vi "Overview.vi"() -> ()   [LabVIEW 2024]
uses:
  <vilib>/Plug-In SDKs/Clients/Metadata/Operator.ctl
  <vilib>/Plug-In SDKs/Clients/Metadata/Extension.ctl
  <vilib>/Plug-In SDKs/Clients/Metadata/Test Station.ctl
  <vilib>/Plug-In SDKs/Clients/Metadata/Software Item.ctl
  <vilib>/Plug-In SDKs/Clients/Data Store V1/Data Store Client.lvlibp/API/Data Store V1/Test Result.ctl
  <vilib>/Plug-In SDKs/Clients/Metadata/Outcome.ctl
  <vilib>/Plug-In SDKs/Clients/Metadata/Step.ctl
  <vilib>/Plug-In SDKs/Clients/Metadata Store V1/Metadata Store Client.lvlibp/API/Metadata Store V1/Register Schema (String).vi
  <vilib>/Plug-In SDKs/Clients/Metadata Store V1/Metadata Store Client.lvlibp/API/Metadata Store V1/Create Operator.vi
  <vilib>/Plug-In SDKs/Clients/Metadata Store V1/Metadata Store Client.lvlibp/API/Metadata Store V1/Create Test Station.vi
  <vilib>/Plug-In SDKs/Clients/Metadata Store V1/Metadata Store Client.lvlibp/API/Metadata Store V1/Create Software Item.vi
  <vilib>/Plug-In SDKs/Clients/Data Store V1/Data Store Client.lvlibp/API/Data Store V1/Publish Measurement (DBL Analog Waveform).vi
  <vilib>/Plug-In SDKs/Clients/Metadata Store V1/Metadata Store Client.lvlibp/API/Metadata Store V1/Get Operator.vi
  <vilib>/Plug-In SDKs/Clients/Data Store V1/Data Store Client.lvlibp/API/Data Store V1/Read Data from Measurement (DBL Analog Waveform).vi
  <vilib>/Plug-In SDKs/Clients/Metadata Store V1/Metadata Store Client.lvlibp
  <vilib>/Plug-In SDKs/Clients/Data Store V1/Data Store Client.lvlibp
  <vilib>/Plug-In SDKs/Clients/Metadata/NI Metadata Types.lvlib
  <vilib>/measure/NI_MABase.lvlib
panel:
  out "test result id":string
  out "published measurement id":string
  out "schema id":string
  out "Waveform Graph":waveform(dbl)(graph)
  out "log":string
  out "error out":errorcluster
  # "This example publishes a waveform along with metadata and metadata extensions.\nThen it queries for the published data and displays it."
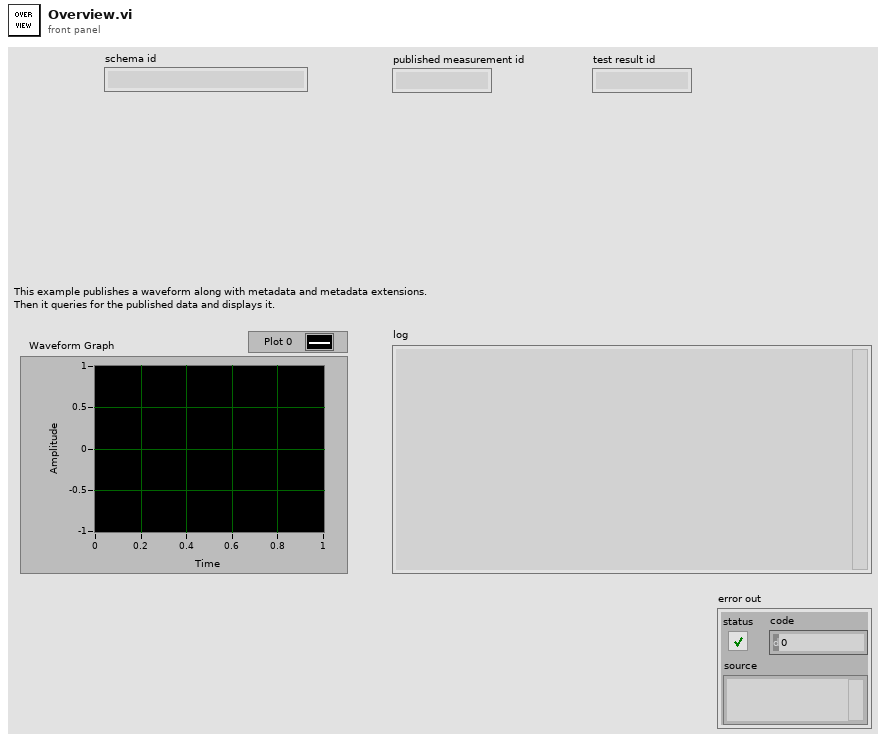
[diagram p1: front panel]
types:
  T1 = enum16{"Register Metadata Schema", "Create Metadata and Test Result", "Publish Data", "Query Published Data"}
  T2 = typedef "NI Metadata Types.lvlib/Extension.ctl" = cluster{"name":string, "value":string}
  T3 = typedef "Data Store Client.lvlibp/Test Result.ctl" = cluster{"test result name":string, "start date time":timestamp, "end date time":timestamp, "outcome":T4, "test result id":string, "uut instance id":string, "operator id":string, "test station id":string, "test description id":string, "software item ids":string[], "hardware item ids":string[], "test adapter ids":string[], "link":string, "extensions":T2[], "schema id":string}
  T4 = typedef "NI Metadata Types.lvlib/Outcome.ctl" = enum32{"Unspecified", "Passed", "Failed", "Indeterminate"}
  T5 = typedef "NI Metadata Types.lvlib/Software Item.ctl" = cluster{"product":string, "version":string, "id":string, "link":string, "extensions":T2[], "schema id":string}
  T6 = typedef "NI Metadata Types.lvlib/Test Station.ctl" = cluster{"test station name":string, "asset identifier":string, "id":string, "link":string, "extensions":T2[], "schema id":string}
  T7 = typedef "NI Metadata Types.lvlib/Operator.ctl" = cluster{"operator name":string, "role":string, "id":string, "link":string, "extensions":T2[], "schema id":string}
  T8 = typedef "NI Metadata Types.lvlib/Step.ctl" = cluster{"step name":string, "step type":string, "start date time":timestamp, "end date time":timestamp, "notes":string, "step id":string, "parent step id":string, "test result id":string, "test id":string, "link":string, "extensions":T2[], "schema id":string}
  T9 = typedef "Data Store Client.lvlibp/Published Measurement.ctl" = cluster{"data moniker":T10, "published conditions":T11[], "published measurement id":string, "test result id":string, "step id":string, "software item ids":string[], "hardware item ids":string[], "test adapter ids":string[], "measurement name":string, "data type":string, "measurement notes":string, "start date time":timestamp, "end date time":timestamp, "outcome":T4, "parametric index":i32, "error information":T12}
  T10 = typedef "Data Store Client.lvlibp/Data Moniker.ctl" = cluster{"service location":string, "data source":string, "data instance":i64}
  T11 = typedef "Data Store Client.lvlibp/Published Condition.ctl" = cluster{"moniker":T10, "published condition id":string, "condition name":string, "condition type":string, "step id":string, "test result id":string}
  T12 = typedef "NI Metadata Types.lvlib/Error Information.ctl" = cluster{"error code":i32, "message":string, "source":string}
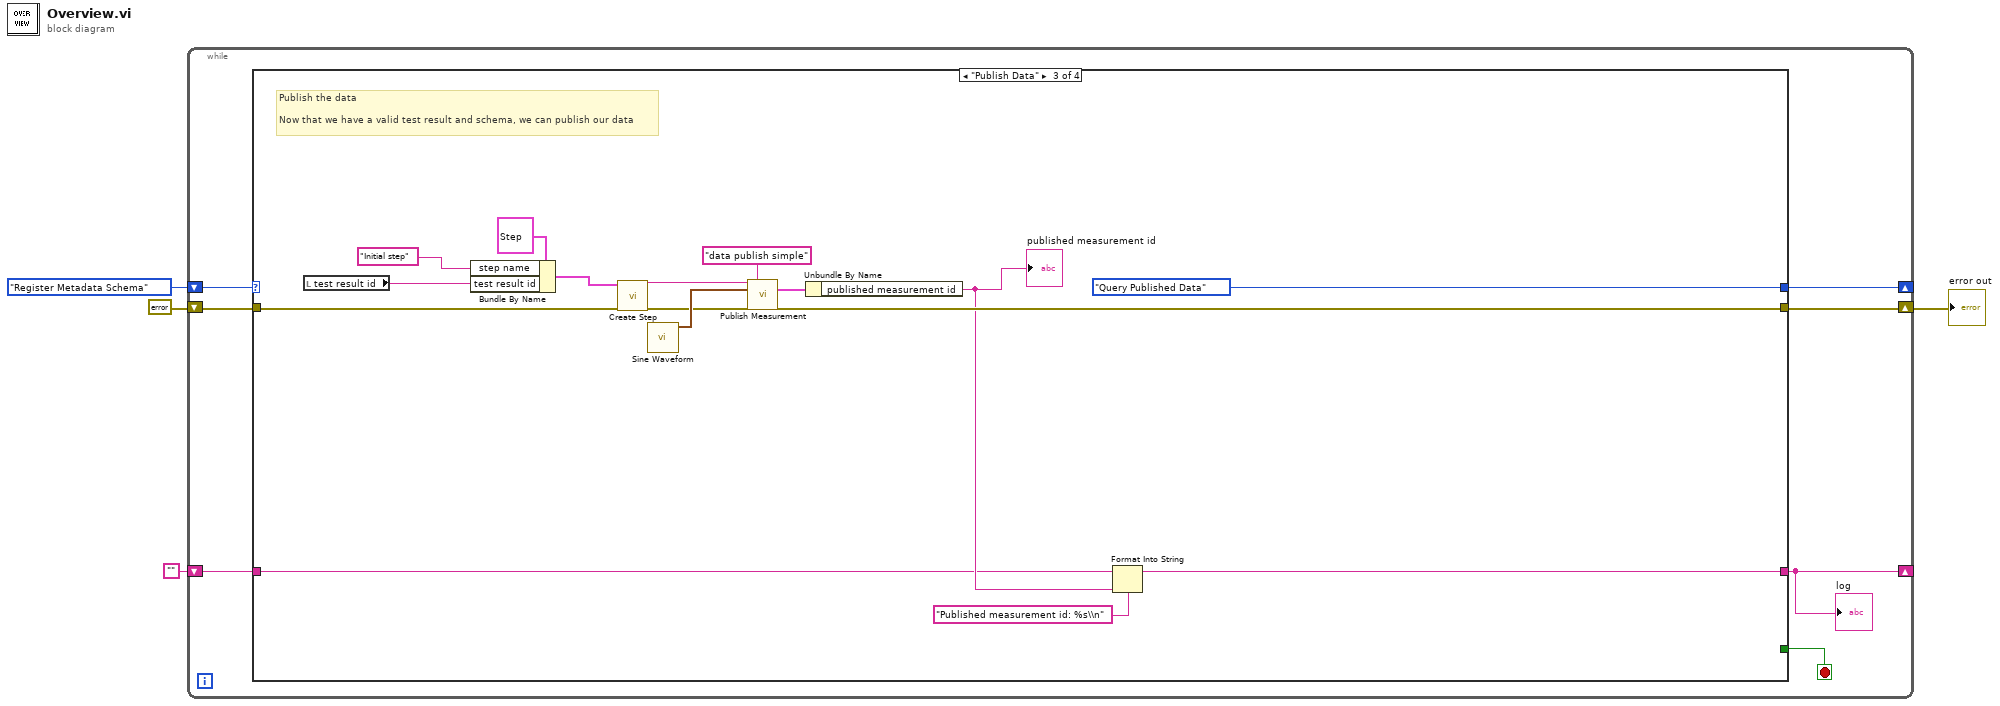
[diagram p0: block diagram]
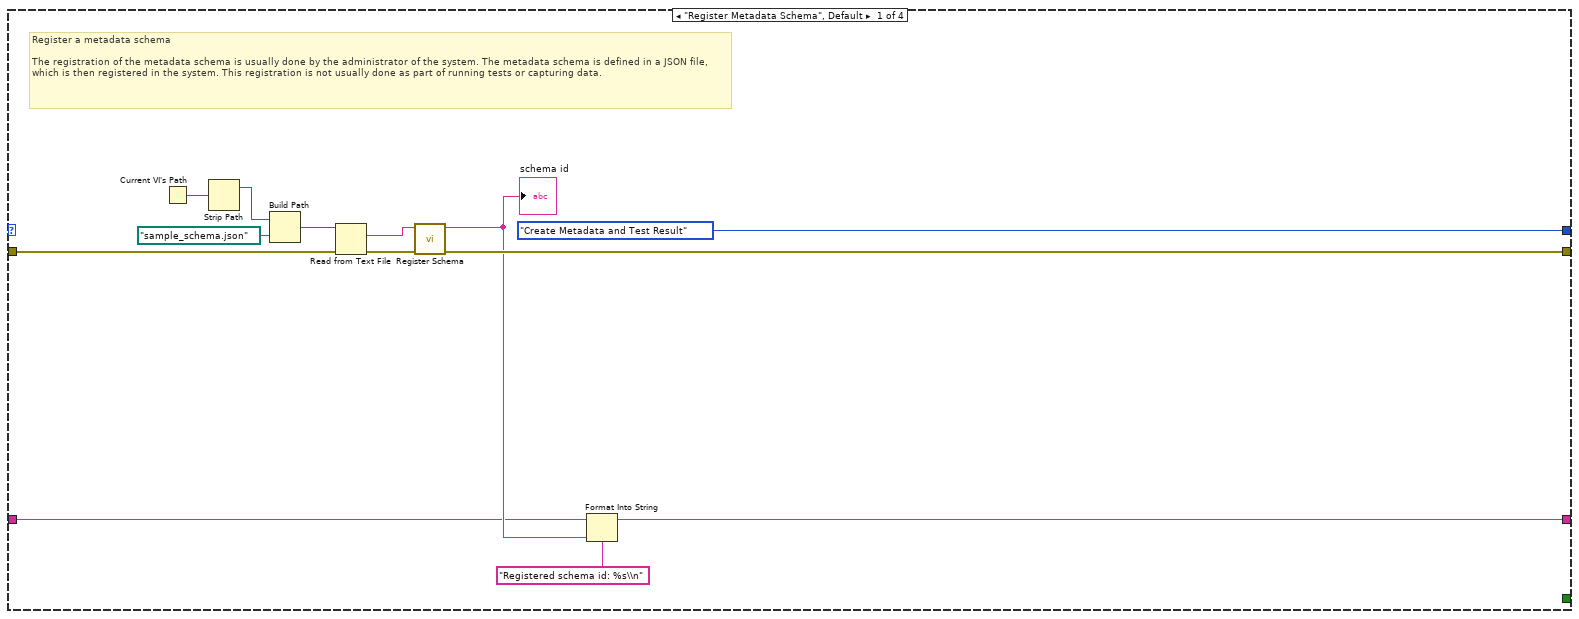
[diagram p2: hidden frame]
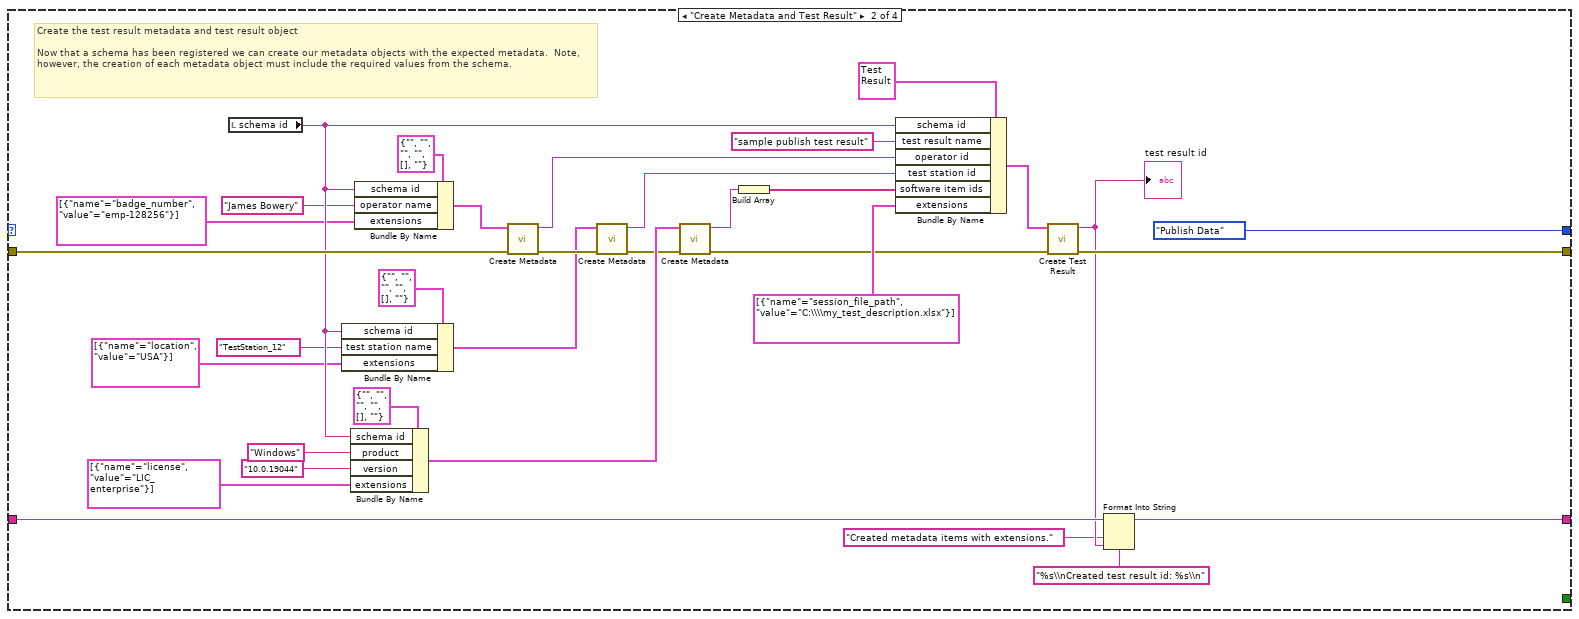
[diagram p3: hidden frame]
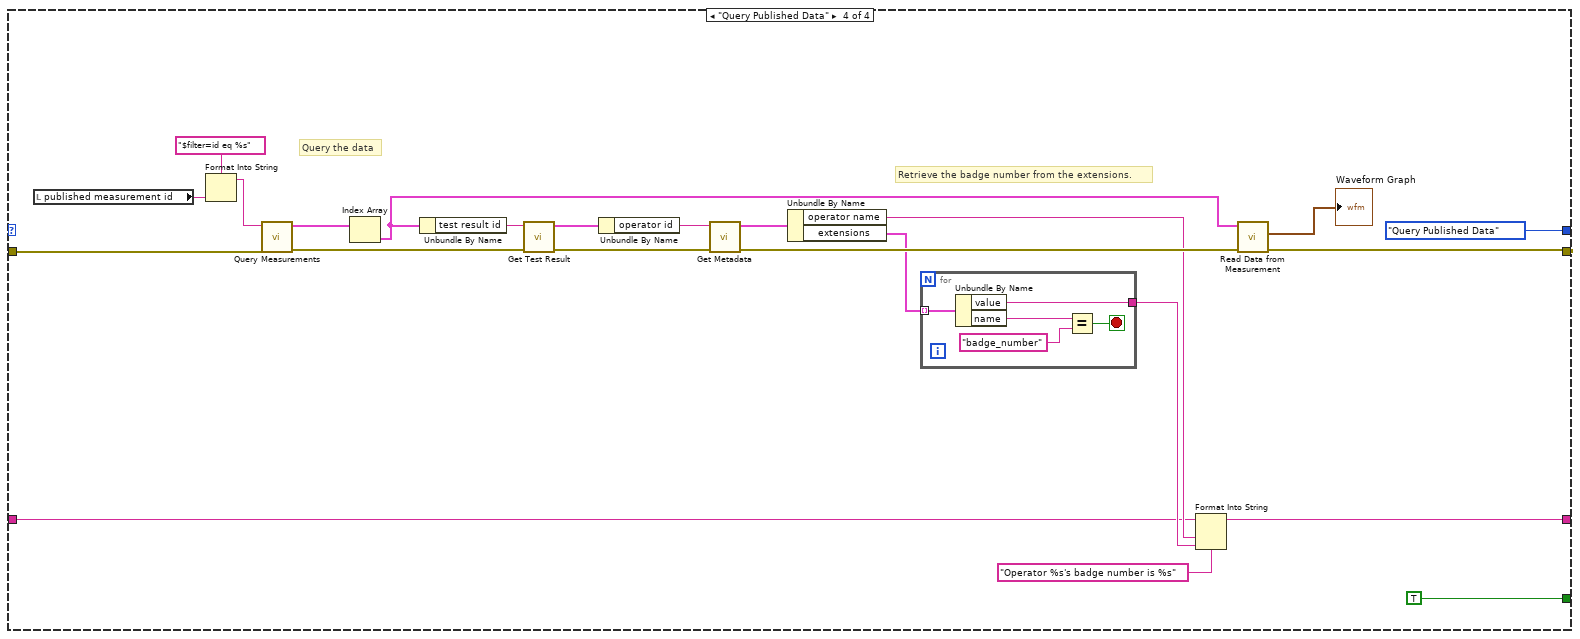
[diagram p4: hidden frame]
diagram:
  n1 = while {
    shift-right: [w7] -> _
    shift-left: T1."Register Metadata Schema" -> [w11]
    shift-right: [w10] -> w2
    shift-left: errorcluster {"status"=FALSE, "code"=0, "source"=""} ("error out") -> [w9]
    shift-right: [w6] -> _
    shift-left: "" ("log") -> [w8]
    stop <- w5 stop-if-true
    n2 = case shown="\"Publish Data\"" w11 {
      tunnel: [w24 w54 w73 w96] -> w10
      tunnel: w9 -> [w23 w55 w61 w95]
      tunnel: [w13 w51 w63 w75] -> w6
      tunnel: w8 -> [w14 w52 w58 w76]
      tunnel: [T1."Create Metadata and Test Result" T1."Publish Data" T1."Query Published Data" T1."Query Published Data"] -> w7
      tunnel: [_ _ _ TRUE] -> w5
      frame "Register Metadata Schema", Default {
        # "Register a metadata schema\n\nThe registration of the metadata schema is usually done by the administrator of the system. The metadata schema is defined in a JSON file, which is then registered in the system. This registration is not usually done as part of running tests or capturing data."
        n3 = Current VI's Path() -> (path=w19:path)
        n4 = Strip Path(path=w19) -> (stripped path=w18:path)  [unwired: 1 out]
        n5 = Build Path(base path=w18, name or relative path=path "sample_schema.json") -> (appended path=w16:path)
        n6 = Read from Text File(file (use dialog)=w16, error in=w23) -> (text=w15:string, error out=w20:errorcluster)  [unwired: 2 in, 2 out]
        n7 = call-poly <vilib>:"Register Schema.vi"("error in"=w20, "schema"=w15) -> ("error out"=w24:errorcluster, "schema id"=w22:string)  [unwired: 8 in]
        "schema id" <- w22
        n8 = Format Into String(format string="Registered schema id: %s\\n", initial string=w14, w22) -> (resulting string=w13:string)  [unwired: 1 in, 1 out]
      }
      frame "Create Metadata and Test Result" {
        # "Create the test result metadata and test result object\n\nNow that a schema has been registered we can create our metadata objects with the expected metadata.  Note, however, the creation of each metadata object must include the required values from the schema."
        n9 = local read "schema id"() -> (w53:string)
        n10 = Bundle By Name(cluster=T6 {"test station name"="", "asset identifier"="", "id"="", "link"="", "extensions"=[], "schema id"=""} ("test station"), "schema id"=w53, "test station name"="TestStation_12", "extensions"=T2[] [{"name"="location", "value"="USA"}]) -> (w25:T6)
        n11 = Bundle By Name(cluster=T5 {"product"="", "version"="", "id"="", "link"="", "extensions"=[], "schema id"=""} ("software item"), "schema id"=w53, "product"="Windows", "version"="10.0.19044", "extensions"=T2[] [{"name"="license", "value"="LIC_enterprise"}]) -> (w29:T5)
        n12 = Bundle By Name(cluster=T7 {"operator name"="", "role"="", "id"="", "link"="", "extensions"=[], "schema id"=""} ("operator metadata"), "schema id"=w53, "operator name"="James Bowery", "extensions"=T2[] [{"name"="badge_number", "value"="emp-128256"}]) -> (w36:T7)
        n13 = call-poly <vilib>:"Create Metadata.vi"("error in"=w55, "operator metadata"=w36) -> ("error out"=w28:errorcluster, "operator id"=w47:string)  [unwired: 8 in]
        n14 = call-poly <vilib>:"Create Metadata.vi"("error in"=w28, "test station"=w25) -> ("error out"=w27:errorcluster, "test station id"=w46:string)  [unwired: 8 in]
        n15 = call-poly <vilib>:"Create Metadata.vi"("error in"=w27, "software item"=w29) -> ("error out"=w26:errorcluster, "software item id"=w45:string)  [unwired: 8 in]
        n16 = Build Array(w45) -> (w42:string[])
        n17 = Bundle By Name(cluster=T3 {"test result name"="", "start date time"=timestamp(0 s since 1904-01-01), "end date time"=timestamp(0 s since 1904-01-01), "outcome"=enum."Unspecified", "test result id"="", "uut instance id"="", "operator id"="", "test station id"="", "test description id"="", "software item ids"=[], "hardware item ids"=[], "test adapter ids"=[], "link"="", "extensions"=[], "schema id"=""} ("test result"), "schema id"=w53, "test result name"="sample publish test result", "operator id"=w47, "test station id"=w46, "software item ids"=w42, "extensions"=T2[] [{"name"="session_file_path", "value"="C:\\\\my_test_description.xlsx"}]) -> (w57:T3)
        n18 = call <vilib>:"Create Test Result.vi"("error in"=w26, "test result"=w57) -> ("error out"=w54:errorcluster, "test result id"=w49:string)  [unwired: 8 in]
        "test result id" <- w49
        n19 = Format Into String(format string="%s\\nCreated test result id: %s\\n", initial string=w52, "Created metadata items with extensions." ("log"), w49) -> (resulting string=w51:string)  [unwired: 1 in, 1 out]
      }
      frame "Publish Data" {
        # "Publish the data\n\nNow that we have a valid test result and schema, we can publish our data"
        n20 = local read "test result id"() -> (w60:string)
        n21 = Bundle By Name(cluster=T8 {"step name"="", "step type"="", "start date time"=timestamp(0 s since 1904-01-01), "end date time"=timestamp(0 s since 1904-01-01), "notes"="", "step id"="", "parent step id"="", "test result id"="", "test id"="", "link"="", "extensions"=[], "schema id"=""} ("step"), "step name"="Initial step", "test result id"=w60) -> (w68:T8)
        n22 = call <vilib>:"Create Step.vi"("error in"=w61, "step"=w68) -> ("error out"=w67:errorcluster, "step id"=w66:string)  [unwired: 8 in]
        n23 = call <vilib>:"Sine Waveform.vi"() -> ("signal out"=w71:waveform(dbl))  [unwired: 10 in, 1 out]
        n24 = call-poly <vilib>:"Publish Measurement.vi"("step id"=w66, "name"="data publish simple", "waveform"=w71, "error in"=w67) -> ("published measurement"=w64:T9, "error out"=w73:errorcluster)  [unwired: 9 in, 1 out]
        n25 = Unbundle By Name(w64) -> ("published measurement id"=w72:string)
        "published measurement id" <- w72
        n26 = Format Into String(format string="Published measurement id: %s\\n", initial string=w58, w72) -> (resulting string=w63:string)  [unwired: 1 in, 1 out]
      }
      frame "Query Published Data" {
        # "Retrieve the badge number from the extensions."
        # "Query the data"
        n27 = local read "published measurement id"() -> (w94:string)
        n28 = Format Into String(format string="$filter=id eq %s", w94) -> (resulting string=w85:string)  [unwired: 2 in, 1 out]
        n29 = call <vilib>:"Query Measurements.vi"("error in"=w95, "odata query"=w85) -> ("error out"=w83:errorcluster, "published measurements"=w84:T9[])  [unwired: 8 in]
        n30 = Index Array(array=w84) -> (element=w77:T9)  [unwired: 1 in]
        n31 = Unbundle By Name(w77) -> ("test result id"=w82:string)
        n32 = call <vilib>:"Get Test Result.vi"("error in"=w83, "test result id"=w82) -> ("error out"=w81:errorcluster, "test result"=w80:T3)  [unwired: 8 in]
        n33 = Unbundle By Name(w80) -> ("operator id"=w79:string)
        n34 = call-poly <vilib>:"Get Metadata.vi"("error in"=w81, "operator id"=w79) -> ("error out"=w91:errorcluster, "operator metadata"=w78:T7)  [unwired: 8 in]
        n35 = Unbundle By Name(w78) -> ("operator name"=w88:string, "extensions"=w89:T2[])
        n36 = for {
          tunnel: w89 -> [w101] mode=indexing
          tunnel: [w97] -> w90
          stop <- w98 stop-if-true
          n37 = Unbundle By Name(w101) -> ("value"=w97:string, "name"=w100:string)
          n38 = Equal?(x=w100, y="badge_number") -> (x = y?=w98:bool)
        }
        n39 = Format Into String(format string="Operator %s's badge number is %s", initial string=w76, w88, w90) -> (resulting string=w75:string)  [unwired: 1 in, 1 out]
        n40 = call-poly <vilib>:"Read Data from Measurement.vi"("error in"=w91, "published measurement"=w77) -> ("error out"=w96:errorcluster, "waveform data"=→"Waveform Graph":waveform(dbl))  [unwired: 7 in, 1 out]
      }
    }
    "log" <- w6
  }
  "error out" <- w2
